vi "pause_time_detector.vi"(7 "timestamp in":u32, 8 "iteration count":i32, 10 "end of message":bool, 11 "incoming character":string) -> (4 "next word":bool, 5 "timestamp out":u32, 6 "next letter":bool)   [LabVIEW 2024]
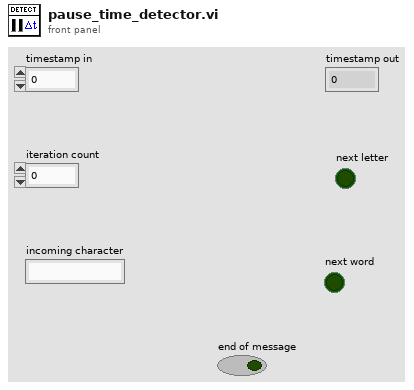
[diagram p1: front panel]
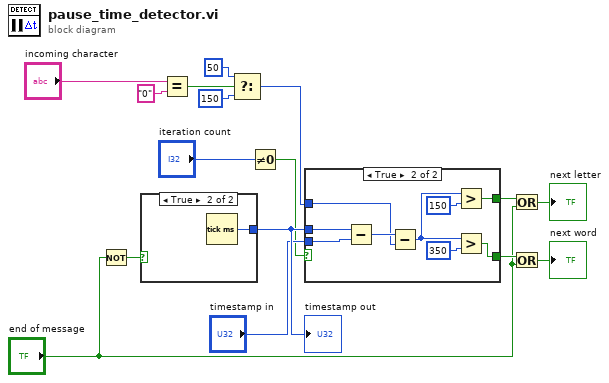
[diagram p0: block diagram]
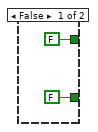
[diagram p2: hidden frame]
diagram:
  n1 = Not(x="end of message") -> (.not. x?=w6:bool)
  n2 = case shown="True" w6 {
    tunnel: [_ w17] -> w15
    frame False {
    }
    frame True {
      n3 = Tick Count (ms)() -> (millisecond timer value=w17:u32)
    }
  }
  "timestamp out" <- w15
  n4 = Equal?(x="incoming character", y="0") -> (x = y?=w8:bool)
  n5 = Select(t=u32 50, s=w8, f=u32 150) -> (s? t:f=w9:u32)
  n6 = Not Equal To 0?(x="iteration count") -> (x != 0?=w12:bool)
  n7 = case shown="True" w12 {
    tunnel: "timestamp in" -> [_ w28]
    tunnel: w15 -> [_ w27]
    tunnel: [FALSE w26] -> w10
    tunnel: w9 -> [_ w24]
    tunnel: [FALSE w23] -> w11
    frame False {
    }
    frame True {
      n8 = Subtract(x=w27, y=w28) -> (x-y=w25:u32)
      n9 = Subtract(x=w25, y=w24) -> (x-y=w22:u32)
      n10 = Greater?(x=w22, y=u32 150) -> (0:w23:bool)
      n11 = Greater?(x=w22, y=u32 350) -> (0:w26:bool)
    }
  }
  n12 = Or(x=w11, y="end of message") -> (x .or. y?=→"next letter":bool)
  n13 = Or(x=w10, y="end of message") -> (x .or. y?=→"next word":bool)
